vi "Calculate DIT.vi"(4 "error in":errorcluster, 5 "DIT Key Info":T1, 6 "Text without DIT":string) -> (0 "error out":errorcluster, 3 "DIT":string)   [LabVIEW 2012]
doc: "Calculates a DIT string based on the inputted Text and Keys. Output is only DIT and does not contain original text."
uses:
  User Access Type defs/DIT Key cluster.ctl
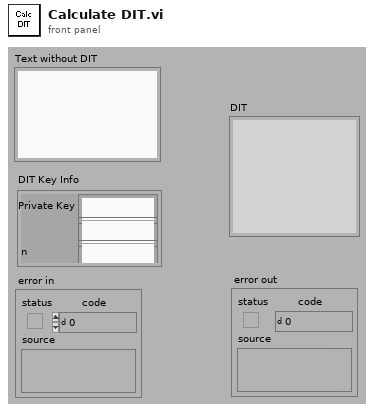
[diagram p1: front panel]
types:
  T1 = typedef "DIT Key cluster.ctl" = cluster{"Private Key":string, "Public Key":string, "n":string}
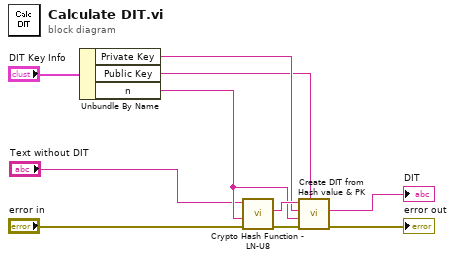
[diagram p0: block diagram]
diagram:
  n1 = Unbundle By Name("DIT Key Info") -> ("Private Key"=w5:string, "Public Key"=w4:string, "n"=w3:string)
  n2 = call "Crypto Hash Function - LN-U8.vi"("error in (no error)"="error in", "n (Hex)"=w3, "Text string"="Text without DIT") -> ("error out"=w7:errorcluster, "Hash value Hex string"=w10:string)  [unwired: 1 in, 6 out]
  n3 = call "Create DIT from Hash value & PK.vi"("Public Key (Hex)"=w4, "error in (no error)"=w7, "n (Hex)"=w3, "Private Key (Hex)"=w5, "Hash value"=w10) -> ("error out"=→"error out":errorcluster, "DIT"=→"DIT":string)  [unwired: 5 out]
